vi "DT_Merge_Stop Check.vi"(9 "Data In":T1, 10 "Triangles In":i32[][](array[numeric]), 11 "Points In":cluster{"x":dbl, "y":dbl, "index":i32}[](array[cluster])) -> (0 "left stop?":bool, 1 "Data Out":T1, 2 "Triangles Out":i32[][](array[numeric]), 3 "Points Out":cluster{"x":dbl, "y":dbl, "index":i32}[](array[cluster]), 4 "right stop?":bool)   [LabVIEW 2017, in "NI_AAL_Geometry.lvlib"]
uses:
  <vilib>/Analysis/NI_AAL_Geometry.lvlib
  <vilib>/Analysis/geometry.llb/DT_Merge_Find Next Triangulation_Data.ctl
  <vilib>/Analysis/geometry.llb/Triangle Area.vi
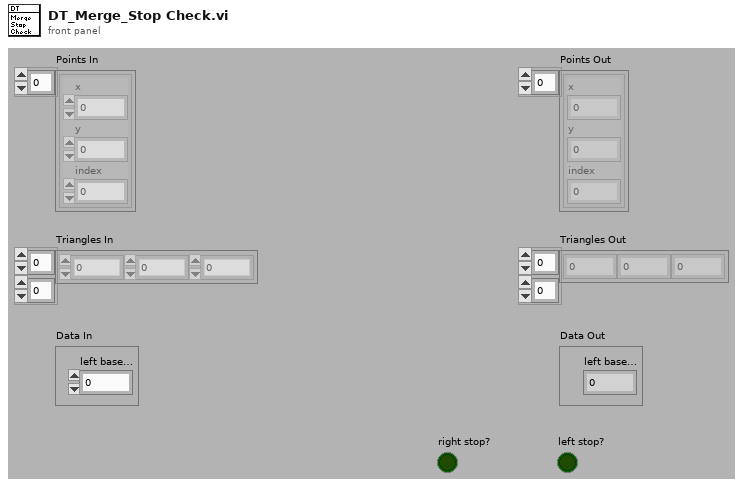
[diagram p1: front panel]
types:
  T1 = typedef "NI_AAL_Geometry.lvlib/DT_Merge_Find Next Triangulation_Data.ctl" = cluster{"left base point":i32, "left triangle":i32, "left local idx":i32, "right base point":i32, "right triangle":i32, "right local idx":i32, "Left Candidate Triangles":i32[], "Left Candidate Point Idx":i32[], "Right Candidate Triangles":i32[], "Right Candidate Point Idx":i32[], "cur triangle":i32}
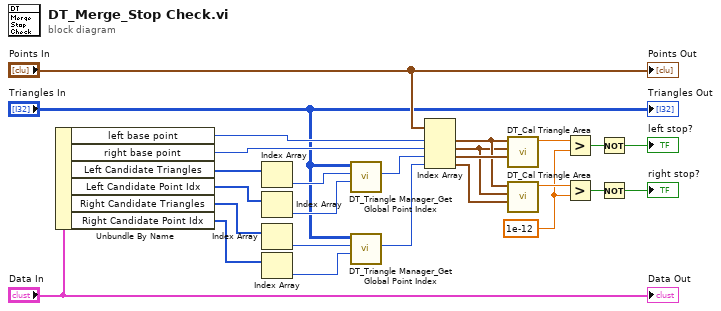
[diagram p0: block diagram]
diagram:
  w13 = 1e-12 ("x")
  n1 = Unbundle By Name("Data In") -> ("left base point"=w2:i32, "right base point"=w3:i32, "Left Candidate Triangles"=w22:i32[], "Left Candidate Point Idx"=w21:i32[], "Right Candidate Triangles"=w18:i32[], "Right Candidate Point Idx"=w17:i32[])
  n2 = Index Array(array=w22) -> (element=w20:i32)  [unwired: 1 in]
  n3 = Index Array(array=w21) -> (element=w19:i32)  [unwired: 1 in]
  n4 = Index Array(array=w18) -> (element=w16:i32)  [unwired: 1 in]
  n5 = Index Array(array=w17) -> (element=w15:i32)  [unwired: 1 in]
  n6 = call <vilib>:"DT_Triangle Manager_Get Global Point Index.vi"("local idx"=w19, "triangle"=w20, "Triangles"="Triangles In") -> ("global idx"=w4:i32)  [unwired: 8 out]
  n7 = call <vilib>:"DT_Triangle Manager_Get Global Point Index.vi"("local idx"=w15, "triangle"=w16, "Triangles"="Triangles In") -> ("global idx"=w5:i32)  [unwired: 8 out]
  n8 = Index Array(array="Points In", index #1=w2, index #2=w3, index #3=w4, index #4=w5) -> (element #1=w10:cluster{"x":dbl, "y":dbl, "index":i32}, element #2=w9:cluster{"x":dbl, "y":dbl, "index":i32}, element #3=w24:cluster{"x":dbl, "y":dbl, "index":i32}, element #4=w8:cluster{"x":dbl, "y":dbl, "index":i32})
  n9 = call <vilib>:"DT_Cal Triangle Area.vi"("p 3"=w24, "p 2"=w9, "p 1"=w10) -> ("area"=w26:dbl)  [unwired: 8 out]
  n10 = call <vilib>:"DT_Cal Triangle Area.vi"("p 3"=w8, "p 2"=w9, "p 1"=w10) -> ("area"=w14:dbl)  [unwired: 8 out]
  n11 = Greater?(x=w26, y=w13) -> (0:w11:bool)
  n12 = Greater?(x=w14, y=w13) -> (0:w7:bool)
  n13 = Not(x=w11) -> (.not. x?=→"left stop?":bool)
  n14 = Not(x=w7) -> (.not. x?=→"right stop?":bool)
  "Points Out" <- "Points In"
  "Triangles Out" <- "Triangles In"
  "Data Out" <- "Data In"
